vi "Pixel Bytes to LED.vi"(8 "error in (no error)":errorcluster, 9 "image":u8[](array[numeric]), 10 "image depth":i32, 11 "Refnum in":refnum<k20>) -> (0 "error out":errorcluster, 2 "LED Data Out":u32[](array[numeric]), 3 "Refnum out":refnum<k20>)   [LabVIEW 2013]
uses:
  <vilib>/Utility/error.llb/Error Cluster From Error Code.vi
  <vilib>/ErrorRing/Error Ring.xnode
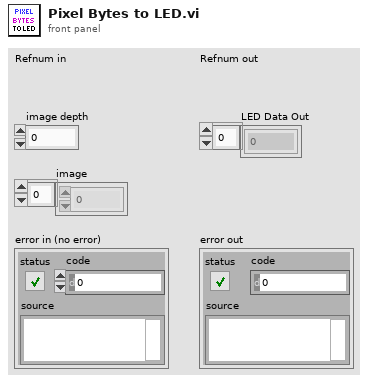
[diagram p1: front panel]
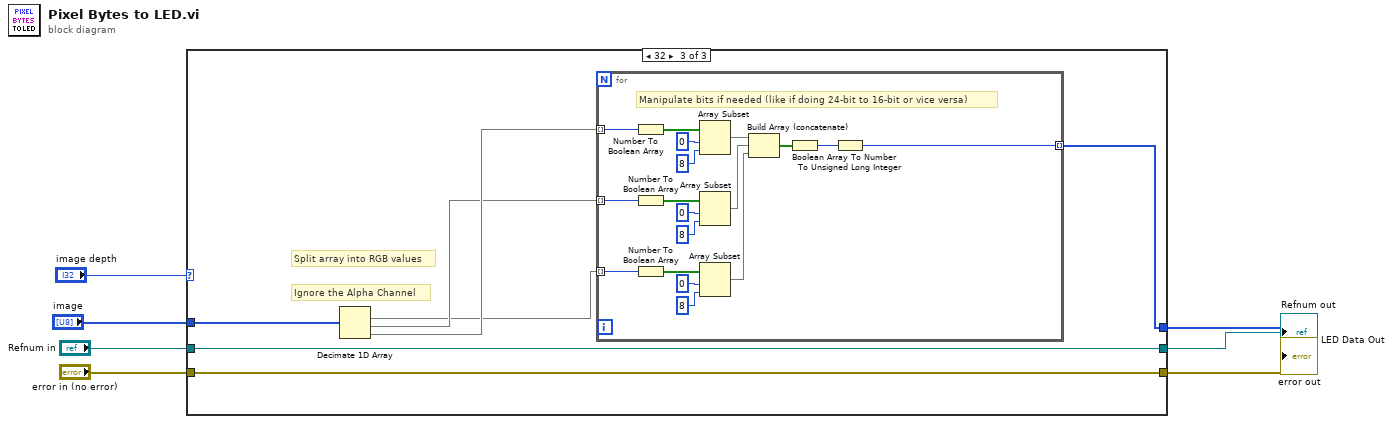
[diagram p0: block diagram]
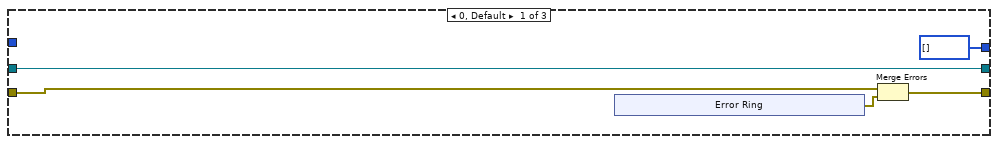
[diagram p2: hidden frame]
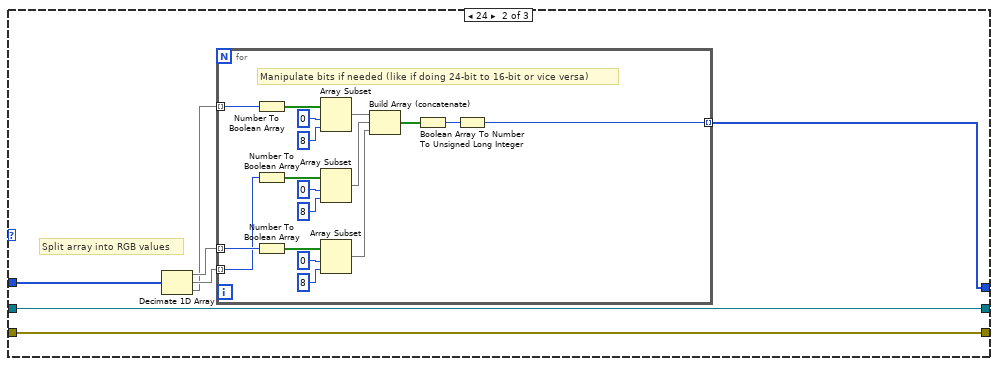
[diagram p3: hidden frame]
diagram:
  n1 = case shown="32" "image depth" {
    tunnel: "error in (no error)" -> [w11 w20 w48]
    tunnel: "image" -> [_ w24 w49]
    tunnel: "Refnum in" -> [w9 w19 w47]
    tunnel: [w12 w20 w48] -> w7
    tunnel: [w9 w19 w47] -> w6
    tunnel: [u32[] [] w18 w46] -> w5
    frame 0, Default {
      n2 = xnode "Error Ring"() -> ("error out"=w10:errorcluster)
      n3 = Merge Errors(w11, w10) -> (w12:errorcluster)
    }
    frame 24 {
      # "Split array into RGB values"
      n4 = Decimate 1D Array(w24) -> (w23:u8[], w22:u8[], w21:u8[])
      n5 = for {
        tunnel: w23 -> [w28] mode=indexing
        tunnel: w22 -> [w27] mode=indexing
        tunnel: w21 -> [w26] mode=indexing
        tunnel: [w25] -> w18 mode=indexing
        # "Manipulate bits if needed (like if doing 24-bit to 16-bit or vice versa)"
        n6 = Number To Boolean Array(number=w26) -> (Boolean array=w34:bool[])
        n7 = Number To Boolean Array(number=w27) -> (Boolean array=w39:bool[])
        n8 = Number To Boolean Array(number=w28) -> (Boolean array=w42:bool[])
        n9 = Array Subset(array=w34, index=0, length=8) -> (w33:bool[])
        n10 = Array Subset(array=w39, index=0, length=8) -> (w32:bool[])
        n11 = Array Subset(array=w42, index=0, length=8) -> (w31:bool[])
        n12 = Build Array (concatenate)(w33, w32, w31) -> (w30:bool[])
        n13 = Boolean Array To Number(Boolean array=w30) -> (number=w29:u32)
        n14 = To Unsigned Long Integer(number=w29) -> (unsigned 32bit integer=w25:u32)
      }
    }
    frame 32 {
      # "Ignore the Alpha Channel"
      # "Split array into RGB values"
      n15 = Decimate 1D Array(w49) -> (w43:u8[], w44:u8[], w45:u8[])  [unwired: 1 out]
      n16 = for {
        tunnel: w43 -> [w53] mode=indexing
        tunnel: w44 -> [w52] mode=indexing
        tunnel: w45 -> [w51] mode=indexing
        tunnel: [w50] -> w46 mode=indexing
        # "Manipulate bits if needed (like if doing 24-bit to 16-bit or vice versa)"
        n17 = Number To Boolean Array(number=w51) -> (Boolean array=w59:bool[])
        n18 = Number To Boolean Array(number=w52) -> (Boolean array=w64:bool[])
        n19 = Number To Boolean Array(number=w53) -> (Boolean array=w67:bool[])
        n20 = Array Subset(array=w59, index=0, length=8) -> (w58:bool[])
        n21 = Array Subset(array=w64, index=0, length=8) -> (w57:bool[])
        n22 = Array Subset(array=w67, index=0, length=8) -> (w56:bool[])
        n23 = Build Array (concatenate)(w58, w57, w56) -> (w55:bool[])
        n24 = Boolean Array To Number(Boolean array=w55) -> (number=w54:u32)
        n25 = To Unsigned Long Integer(number=w54) -> (unsigned 32bit integer=w50:u32)
      }
    }
  }
  "error out" <- w7
  "Refnum out" <- w6
  "LED Data Out" <- w5
